vi "PID cRIO test.vi"() -> ()   [LabVIEW 2021]
panel:
  in  "cRIO IP":string="//172.22.11.2"
  out "error out":errorcluster
  in  "error in (no error)":errorcluster
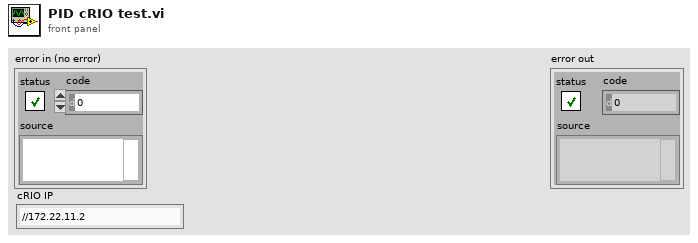
[diagram p1: front panel]
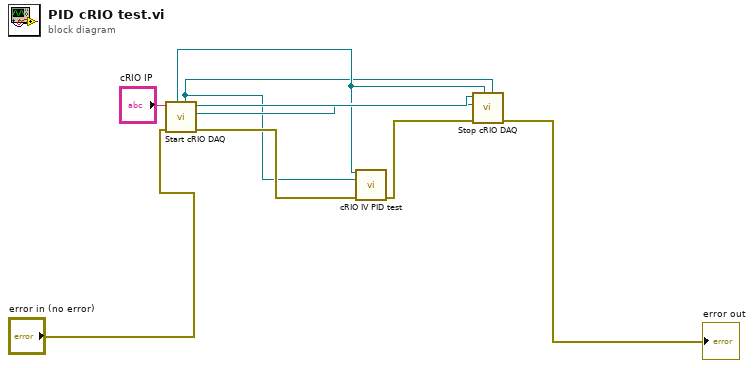
[diagram p0: block diagram]
diagram:
  n1 = call "Start cRIO DAQ.vi"("error in (no error)"="error in (no error)", "cRIO IP"="cRIO IP") -> ("error out"=w7:errorcluster, "vi reference"=w5:refnum<vi>, "application reference"=w6:refnum<vi>, "DAQ_AI_Reader endpoint"=w3:refnum<k21>, "DAQ_CMD_Writer endpoint"=w4:refnum<k21>)  [unwired: 5 in]
  n2 = call "cRIO IV PID test.vi"(0:w4, 5:w3, 11:w7) -> ("error out"=w2:errorcluster)  [unwired: 11 in, 1 out]
  n3 = call "Stop cRIO DAQ.vi"("DAQ_AI_Reader endpoint"=w3, "DAQ_CMD_Writer endpoint"=w4, "error in (no error)"=w2, "VI reference"=w5, "application reference"=w6) -> ("error out"=→"error out":errorcluster)  [unwired: 6 in]
